vi "setPower.vi"(8 "error in (no error)":errorcluster, 9 "Channel":i32, 10 "Power (dBm)":dbl, 11 "Instrument.VSource in":refnum<class "Instrument.VNA.lvclass">) -> (0 "error out":errorcluster, 3 "Instrument.VSource out":refnum<class "Instrument.VNA.lvclass">)   [LabVIEW 2019, in "Instrument.VNA.lvclass"]
uses:
  Instrument.VNA.lvclass
  C:/Users/patrick/Documents/GitHub/Instrument-Framework/lvsrc/Instrument/Instrument.lvclass
  Typedefs/setPower--cluster.ctl
  74b36511-83a5-4780-a8bc-068746ed8036.vi
  74b36511-83a5-4780-a8bc-068746ed8036.vi/f9f6b34b-e377-4372-87c6-17fefd957b0b.vi
  74b36511-83a5-4780-a8bc-068746ed8036.vi/f9f6b34b-e377-4372-87c6-17fefd957b0b.vi/e433e51d-30ef-4d8c-9ceb-594ed2e01cc2.vi
  74b36511-83a5-4780-a8bc-068746ed8036.vi/f9f6b34b-e377-4372-87c6-17fefd957b0b.vi/ad036417-9198-4196-9c7f-46787c882717.vi
  Instrument/Private/Get RC Connection Status.vi
  Instrument/API/Send and Receive.vi
  <vilib>/Utility/Data Type/Get Type Information.vi
  <vilib>/JDP Science/JSONtext/JSON text to Variant.vi
  <vilib>/JDP Science/JSONtext/LVClass Serializer/JSONtext LVClass Serializer.lvclass
  Instrument/Instrument.lvclass
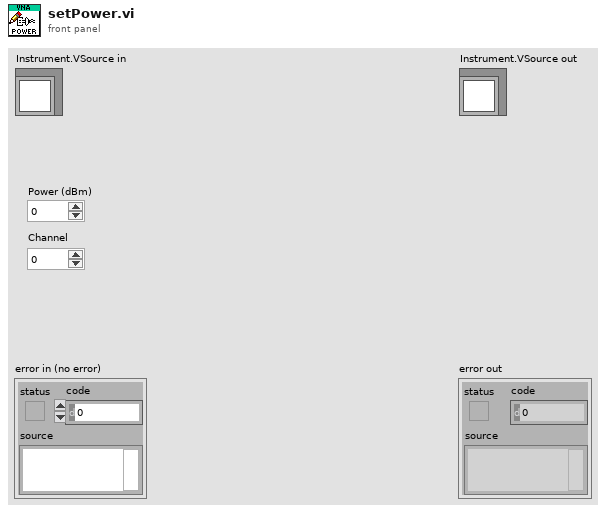
[diagram p1: front panel]
types:
  T1 = typedef "Instrument.VNA.lvclass/setPower--cluster.ctl" = cluster{"power":dbl, "channel":i32}
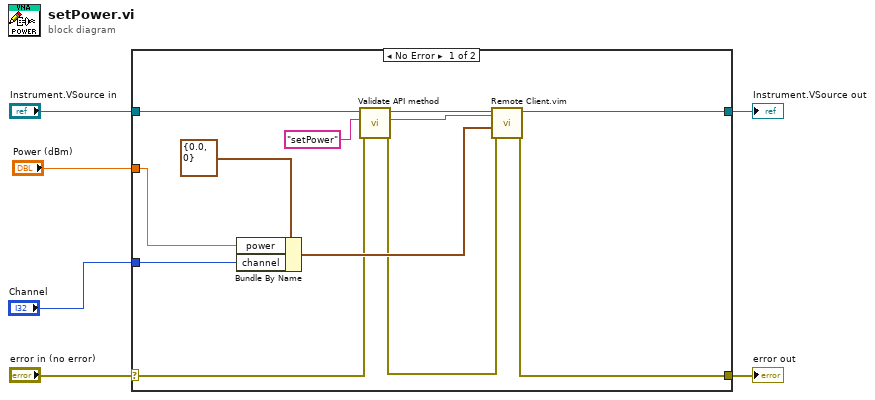
[diagram p0: block diagram]
diagram:
  n1 = case shown="No Error" "error in (no error)" {
    selector: "error in (no error)" -> [w10 w20]
    tunnel: [w8 w20] -> w5
    tunnel: [w14 w19] -> w3
    tunnel: "Instrument.VSource in" -> [w15 w19]
    tunnel: "Power (dBm)" -> [w12 _]
    tunnel: "Channel" -> [w11 _]
    frame No Error {
      n2 = Bundle By Name(cluster=T1 {"power"=0.0, "channel"=0} ("setPower"), "power"=w12, "channel"=w11) -> (w16:T1)
      n3 = call "Validate API method.vi"("error in (no error)"=w10, "Command in"="setPower" ("error message (\"\")"), "Instrument in"=w15) -> ("error out"=w9:errorcluster, "command out"=w17:string, "Instrument out"=w7:refnum<class "Instrument.VNA.lvclass">)  [unwired: 6 in]
      n4 = call "Remote Client.vim"("Data Out type"=w17, "error in (no error)"=w9, "Data in"=w16, "Instrument in"=w7) -> ("error out"=w8:errorcluster, "Instrument out"=w14:refnum<class "Instrument.VNA.lvclass">)  [unwired: 4 in, 2 out]
    }
    frame Error {
    }
  }
  "error out" <- w5
  "Instrument.VSource out" <- w3
